vi "update_two_array_attribute_cmdlist.vi"(5 "Add to Cmd Pool":refnum<vi>, 7 "Delete from Cmd Pool":refnum<vi>, 9 "Modified Array":i32[](array[numeric])) -> ()   [LabVIEW 2018]
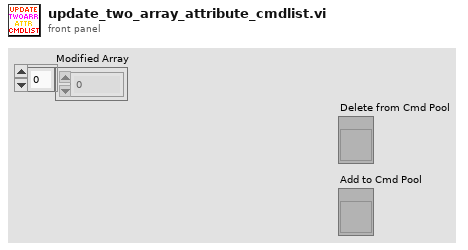
[diagram p1: front panel]
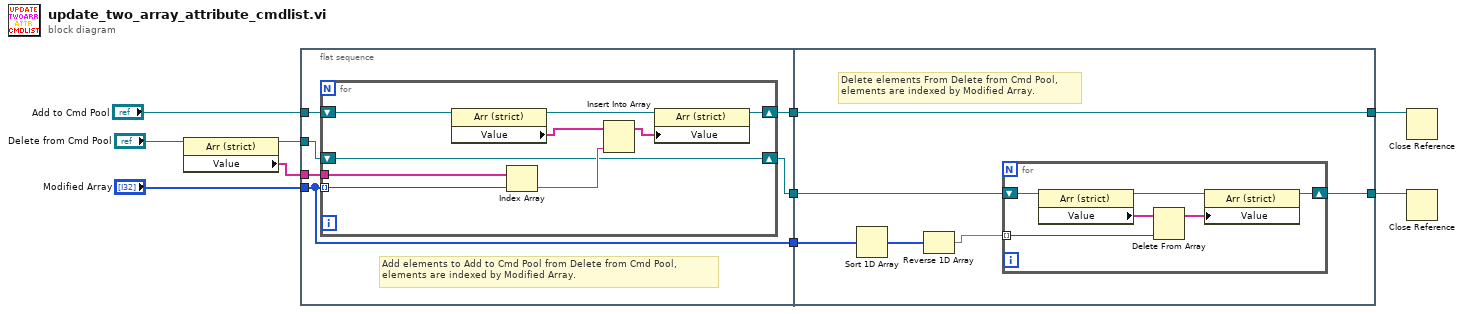
[diagram p0: block diagram]
diagram:
  n1 = property class="Arr (strict)"(reference="Delete from Cmd Pool") -> (reference out=w3:refnum<vi>, "Value"=w6:string[])  [unwired: 1 in, 1 out]
  n2 = flat-sequence {
    tunnel: "Add to Cmd Pool" -> [w15]
    tunnel: "Modified Array" -> [w11]
    tunnel: [w16] -> w10
    tunnel: [w14] -> w9
    tunnel: w3 -> [w13]
    tunnel: w6 -> [w12]
    tunnel: [w11] -> w5
    tunnel: w10 -> [w31]
    tunnel: w9 -> [w29]
    tunnel: w5 -> [w27]
    tunnel: [w29] -> w2
    tunnel: [w28] -> w1
    frame #0 {
      # "Add elements to Add to Cmd Pool from Delete from Cmd Pool,\nelements are indexed by Modified Array."
      n3 = for {
        tunnel: w11 -> [w22] mode=indexing
        tunnel: w12 -> [w17]
        shift-right: [w23] -> w14
        shift-left: w15 -> [w21]
        shift-right: [w18] -> w16
        shift-left: w13 -> [w18]
        n4 = property class="Arr (strict)"(reference=w21) -> (reference out=w19:refnum<vi>, "Value"=w20:string[])  [unwired: 1 in, 1 out]
        n5 = Index Array(array=w17, index=w22) -> (element=w25:string)
        n6 = Insert Into Array(array=w20, new element=w25) -> (w24:string[])  [unwired: 1 in]
        n7 = property class="Arr (strict)"(reference=w19, "Value"=w24) -> (reference out=w23:refnum<vi>)  [unwired: 1 in, 1 out]
      }
    }
    frame #1 {
      # "Delete elements From Delete from Cmd Pool,\nelements are indexed by Modified Array."
      n8 = Sort 1D Array(array=w27) -> (sorted array=w26:i32[])
      n9 = Reverse 1D Array(array=w26) -> (reversed array=w30:i32[])
      n10 = for {
        tunnel: w30 -> [w32] mode=indexing
        shift-right: [w37] -> w28
        shift-left: w31 -> [w33]
        n11 = property class="Arr (strict)"(reference=w33) -> (reference out=w36:refnum<vi>, "Value"=w34:string[])  [unwired: 1 in, 1 out]
        n12 = Delete From Array(array=w34, index=w32) -> (array with subset deleted=w35:string[])  [unwired: 1 in, 1 out]
        n13 = property class="Arr (strict)"(reference=w36, "Value"=w35) -> (reference out=w37:refnum<vi>)  [unwired: 1 in, 1 out]
      }
    }
  }
  n14 = Close Reference(reference=w2) -> ()  [unwired: 1 in, 1 out]
  n15 = Close Reference(reference=w1) -> ()  [unwired: 1 in, 1 out]
